vi "AnalyzeStaticLinkages.vi"(0 "LabVIEW File to Analyze":path, 5 "Public Server Directory":path, 11 "error in":errorcluster) -> (15 "error out":errorcluster)   [LabVIEW 2013, in "LinksApplication.lvclass"]
uses:
  LinksApplication.lvclass
  Featherweight/Core/JSON/FTW-JSON-Escape.vi
panel:
  out "Progress":string
  # "Inputs"
  # "Debug"
  # "Outputs"
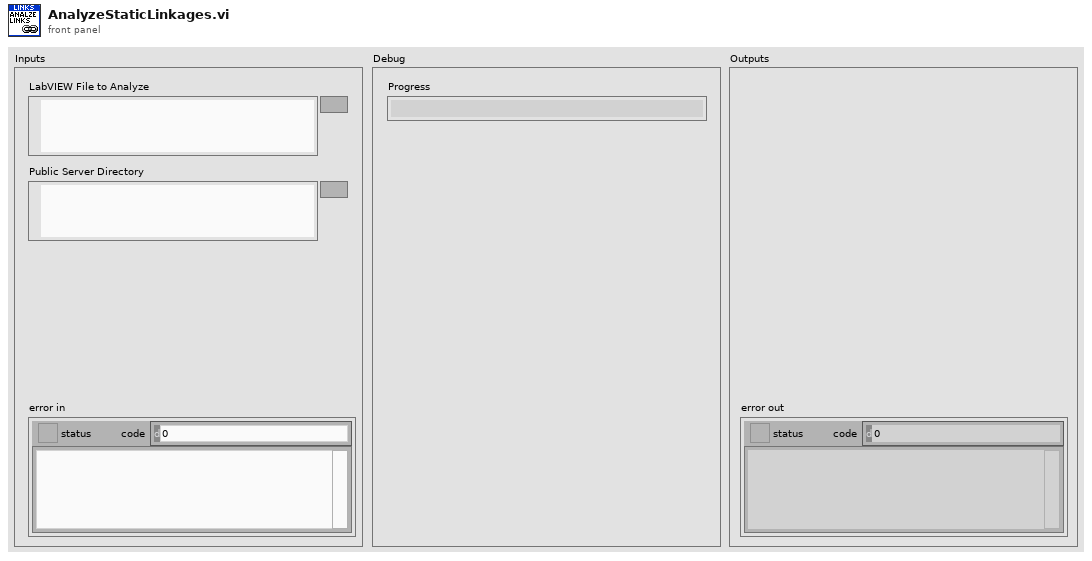
[diagram p1: front panel]
types:
  T1 = cluster{"name":string, "owner":string, "collapsible":bool, "canOpen":bool, "isReentrant":bool, "isInlined":bool}
  T2 = cluster{"nodes":cluster{"name":string, "owner":string, "collapsible":bool, "canOpen":bool, "isReentrant":bool, "isInlined":bool}[], "links":cluster{"source":i32, "target":u32, "value":i32}[]}
  T3 = enum32{"invalid app kind", "Development System", "Run Time System", "Student Edition", "Embedded LabVIEW", "Evaluation", "Custom"}
  T4 = typedef "FTW-Linker-LinkerInfoStructure.ctl" = cluster{"path":path, "delimited name":string, "Filetype":T5, "iState":u32, "iStyle":u16, "wStyle":u16, "buttons":u16, "viflags":u32, "viflags2":u32, "links":u32[]}
  T5 = typedef "FTW-Linker-LabVIEWFiletype.ctl" = enum32{"Invalid file", "Unknown type", "Instrument", "Control", "Polymorphic VI", "Project", "Library", "LVClass", "XControl", "XNode", "Shared library", ".NET assembly", "ActiveX interface", "CIN", "Run-time menu", "Palette menu", "Help file", "LLB", "XNode Edit Dependency", "Class Private Data Control", "Statechart", "MathScript .m file", "Ladder Diagram", "LVLibp", "XNode Build Dependency"}
  T6 = typedef "imagedata.ctl" = cluster{"image type":i32, "image depth":i32, "image":u8[], "mask":u8[], "colors":u32[], "Rectangle":cluster{"left":i16, "top":i16, "right":i16, "bottom":i16}}
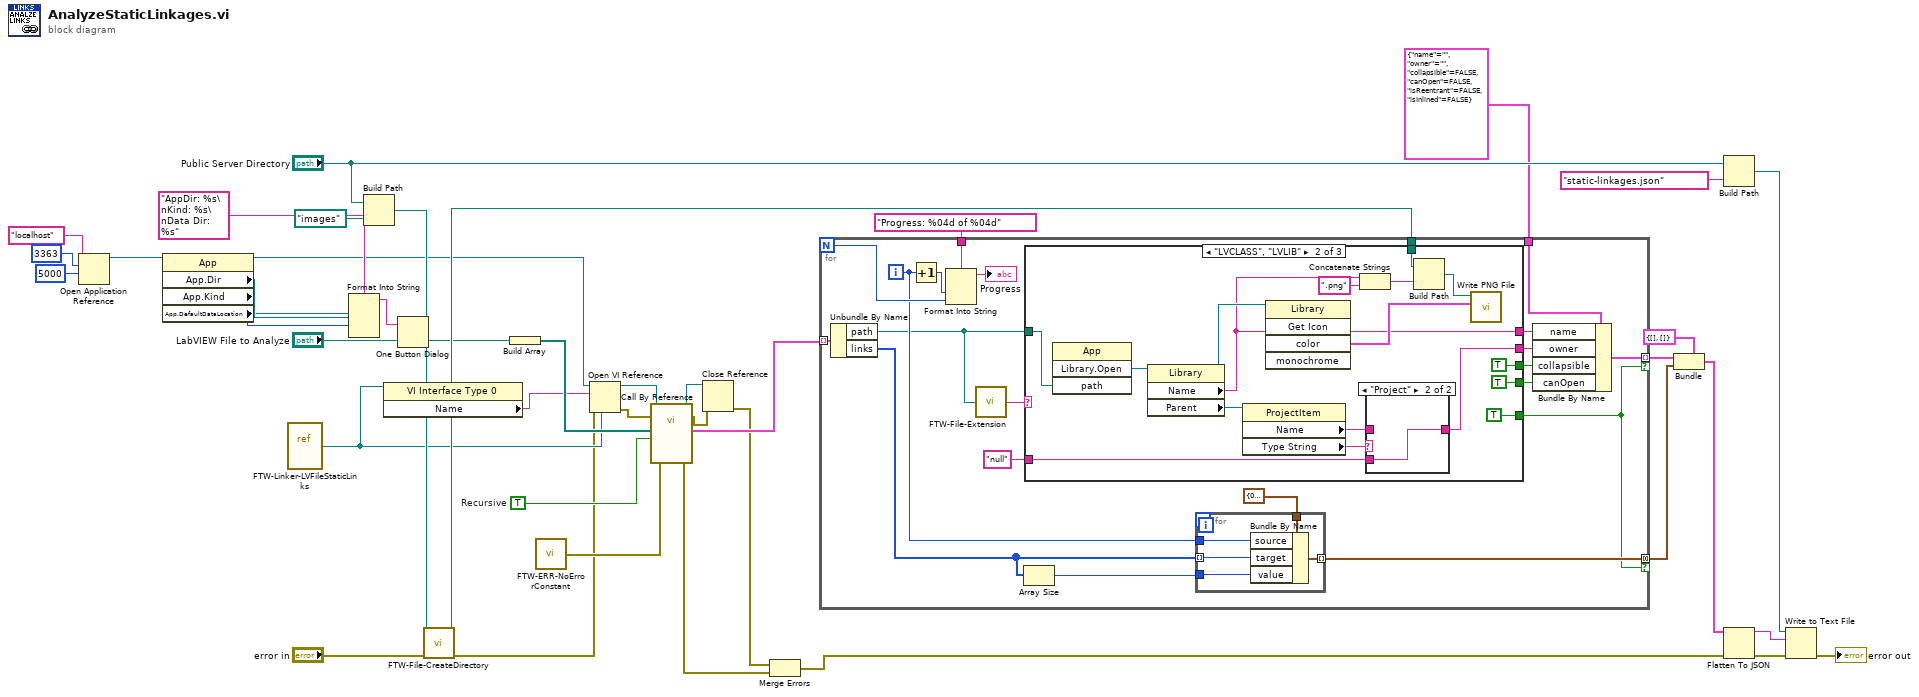
[diagram p0: block diagram]
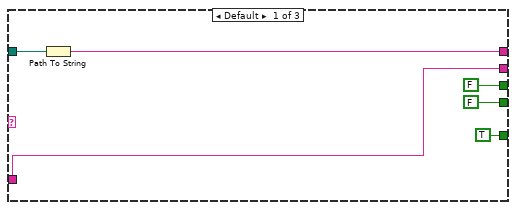
[diagram p2: hidden frame]
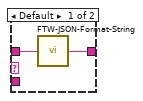
[diagram p3: hidden frame]
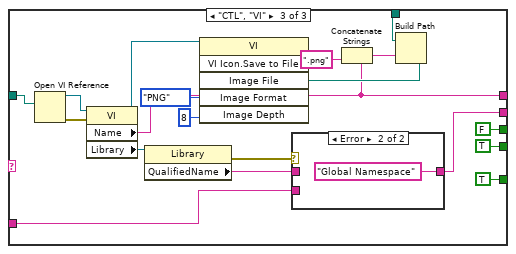
[diagram p4: hidden frame]
diagram:
  w19 = TRUE  # Recursive
  n1 = Open Application Reference(9:5000 ("timeout ms (60000)"), 10:u16 3363 ("port number or service name (3363)"), 11:"localhost" ("machine name (\"\":  open local reference)")) -> (3:w9:refnum<vi>)  [unwired: 1 in, 1 out]
  n2 = property class="App"(reference=w9) -> (reference out=w3:refnum<vi>, "App.Dir"=w7:path, "App.Kind"=w5:T3, "App.DefaultDataLocation"=w4:path)  [unwired: 1 in, 1 out]
  n3 = vi-ref "FTW-Linker-LVFileStaticLinks.vi"() -> (w14:refnum<vi>)
  n4 = Format Into String(format string="AppDir: %s\nKind: %s\nData Dir: %s", w7, w5, w4) -> (resulting string=w8:string)  [unwired: 2 in, 1 out]
  n5 = Build Path(base path="Public Server Directory", name or relative path=path "images") -> (appended path=w36:path)
  n6 = property class="VI Interface Type 0"(reference=w14) -> ("Name"=w13:string)  [unwired: 1 in, 2 out]
  n7 = One Button Dialog(message=w8) -> ()  [unwired: 1 in, 1 out]
  n8 = call "FTW-File-CreateDirectory.vi"("Directory to Create"=w36, "error in"="error in") -> ("Created Directory"=w35:path, "error out"=w11:errorcluster)  [unwired: 12 in]
  n9 = Build Array("LabVIEW File to Analyze") -> (w23:path[])
  n10 = call "FTW-ERR-NoErrorConstant.vi"() -> ("no error"=w15:errorcluster)
  n11 = Open VI Reference(type specifier VI Refnum (for type only)=w14, application reference (local)=w3, vi path=w13, error in (no error)=w11) -> (vi reference=w24:refnum<vi>, error out=w10:errorcluster)  [unwired: 2 in]
  n12 = call-by-ref "?"(reference=w24, error in=w10, "error in"=w15, "Recursive"=w19, "LabVIEW Files"=w23) -> (reference out=w18:refnum<vi>, error out=w17:errorcluster, 0:"error out"=w21:errorcluster, "LinkerInfo"=w22:T4[])  [unwired: 7 in]
  n13 = Close Reference(reference=w18, error in (no error)=w17) -> (error out=w16:errorcluster)
  n14 = Merge Errors(w16, w21) -> (w20:errorcluster)
  n15 = for {
    N -> [w60]
    tunnel: w22 -> [w62] mode=indexing
    tunnel: [w50] -> w34 mode=indexing if=w46
    tunnel: "Progress: %04d of %04d" -> [w61]
    tunnel: [w58] -> w33 mode=concatenating if=w46
    tunnel: w35 -> [w51]
    tunnel: T1 {"name"="", "owner"="", "collapsible"=FALSE, "canOpen"=FALSE, "isReentrant"=FALSE, "isInlined"=FALSE} -> [w42]
    i -> [w55]
    n16 = Unbundle By Name(w62) -> ("path"=w54:path, "links"=w57:u32[])
    n17 = Increment(x=w55) -> (x+1=w59:i32)
    n18 = Format Into String(format string=w61, w59, w60) -> (resulting string=→"Progress":string)  [unwired: 2 in, 1 out]
    n19 = call "FTW-File-Extension.vi"("Filepath"=w54) -> ("Extension"=w53:string)
    n20 = Array Size(array=w57) -> (size(s)=w56:i32)
    n21 = case shown="\"LVCLASS\", \"LVLIB\"" w53 {
      tunnel: w54 -> [w73 w90 w112]
      tunnel: [w72 w80 w97] -> w45
      tunnel: [w71 w85 w106] -> w49
      tunnel: "null" ("QualifiedName") -> [w71 w84 w105]
      tunnel: w51 -> [_ w77 w99]
      tunnel: [FALSE TRUE FALSE] -> w48
      tunnel: [FALSE TRUE TRUE] -> w47
      tunnel: [TRUE TRUE TRUE] -> w46
      frame Default {
        n22 = Path To String(path=w73) -> (string=w72:string)
      }
      frame "LVCLASS", "LVLIB" {
        n23 = invoke class="App" method="Library.Open"("path"=w90) -> ("Open Library"=w89:refnum<vi>)  [unwired: 3 in, 3 out]
        n24 = property class="Library"(reference=w89) -> (reference out=w83:refnum<vi>, "Name"=w80:string, "Parent"=w88:refnum<vi>)  [unwired: 1 in, 1 out]
        n25 = property class="ProjectItem"(reference=w88) -> ("Name"=w86:string, "Type String"=w87:string)  [unwired: 1 in, 2 out]
        n26 = invoke class="Library" method="Get Icon"(reference=w83) -> ("color"=w82:T6)  [unwired: 4 in, 4 out]
        n27 = Concatenate Strings(w80, ".png" ("string")) -> (w78:string)
        n28 = case shown="\"Project\"" w87 {
          tunnel: w86 -> [w92 _]
          tunnel: [w91 w93] -> w85
          tunnel: w84 -> [_ w93]
          frame Default {
            n29 = call "FTW-JSON-Format-String.vi"("LabVIEW String"=w92) -> ("JSON String"=w91:string)
          }
          frame "Project" {
          }
        }
        n30 = Build Path(base path=w77, name or relative path=w78) -> (appended path=w79:path)
        n31 = call <vilib>:"Write PNG File.vi"("image data"=w82, "path to PNG file"=w79) -> ()  [unwired: 8 in, 2 out]
      }
      frame "CTL", "VI" {
        n32 = Open VI Reference(vi path=w112) -> (vi reference=w111:refnum<vi>, error out=w110:errorcluster)  [unwired: 5 in]
        n33 = property class="VI"(reference=w111, error in=w110) -> (reference out=w102:refnum<vi>, "Name"=w97:string, "Library"=w109:refnum<vi>)  [unwired: 1 out]
        n34 = property class="Library"(reference=w109) -> (error out=w108:errorcluster, "QualifiedName"=w107:string)  [unwired: 1 in, 1 out]
        n35 = case shown="Error" w108 {
          tunnel: w107 -> [w113 _]
          tunnel: [w113 "Global Namespace" ("JSON String")] -> w106
          tunnel: w105 -> [_ _]
          frame No Error {
          }
          frame Error {
          }
        }
        n36 = Concatenate Strings(w97, ".png" ("string")) -> (w103:string)
        n37 = Build Path(base path=w99, name or relative path=w103) -> (appended path=w98:path)
        n38 = invoke class="VI" method="VI Icon.Save to File"(reference=w102, "Image File"=w98, "Image Format"=enum32{"PNG", "JPEG", "GIF", "BMP"}."PNG", "Image Depth"=8) -> ()  [unwired: 2 in, 6 out]
      }
    }
    n39 = for {
      tunnel: w57 -> [w66] mode=indexing
      tunnel: w55 -> [w67]
      tunnel: [w64] -> w58 mode=indexing
      tunnel: w56 -> [w65]
      tunnel: cluster{"source":i32, "target":u32, "value":i32} {"source"=0, "target"=0, "value"=0} -> [w63]
      n40 = Bundle By Name(cluster=w63, "source"=w67, "target"=w66, "value"=w65) -> (w64:cluster{"source":i32, "target":u32, "value":i32})
    }
    n41 = Bundle By Name(cluster=w42, "name"=w45, "owner"=w49, "collapsible"=w48, "canOpen"=w47) -> (w50:T1)
  }
  n42 = Bundle(cluster=T2 {"nodes"=[], "links"=[]}, "nodes"=w34, "links"=w33) -> (w31:T2)
  n43 = Build Path(base path="Public Server Directory", name or relative path="static-linkages.json" ("Object Key")) -> (appended path=w39:path)
  n44 = Flatten To JSON(anything=w31, error in (no error)=w20) -> (JSON string=w38:string, 11:w30:errorcluster)  [unwired: 1 in]
  n45 = Write to Text File(file (use dialog)=w39, text=w38, error in=w30) -> (error out=→"error out":errorcluster)  [unwired: 1 in, 2 out]
